vi "Tag_settings_load.vi"(8 "error in (no error)":errorcluster, 10 "PresetName":string, 11 "Gviewer in":refnum<class "Gviewer.lvclass">) -> (0 "error out":errorcluster, 3 "Gviewer out":refnum<class "Gviewer.lvclass">)   [LabVIEW 2020, in "Sgraph_lib_V1.lvlib" / "Gviewer.lvclass"]
doc: "Andre Koelewijn, 5 feb 2021\n\nLoad presets for one of the Viewports"
uses:
  Gviewer.lvclass
  controls/Typedef-PresetFileFormat.ctl
  controls/EditTagOneTag.ctl
  Gviewer.lvclass/Gviewer.ctl
  controls/Typedef_SelProperties.ctl
  controls/Typedef_LineType.ctl
  controls/Typedef_Live.ctl
panel:
  out "value":T1 {"PresetSave"."Presets"."max" format="%#_3p"; "PresetSave"."Presets"."min" format="%#_3p"}
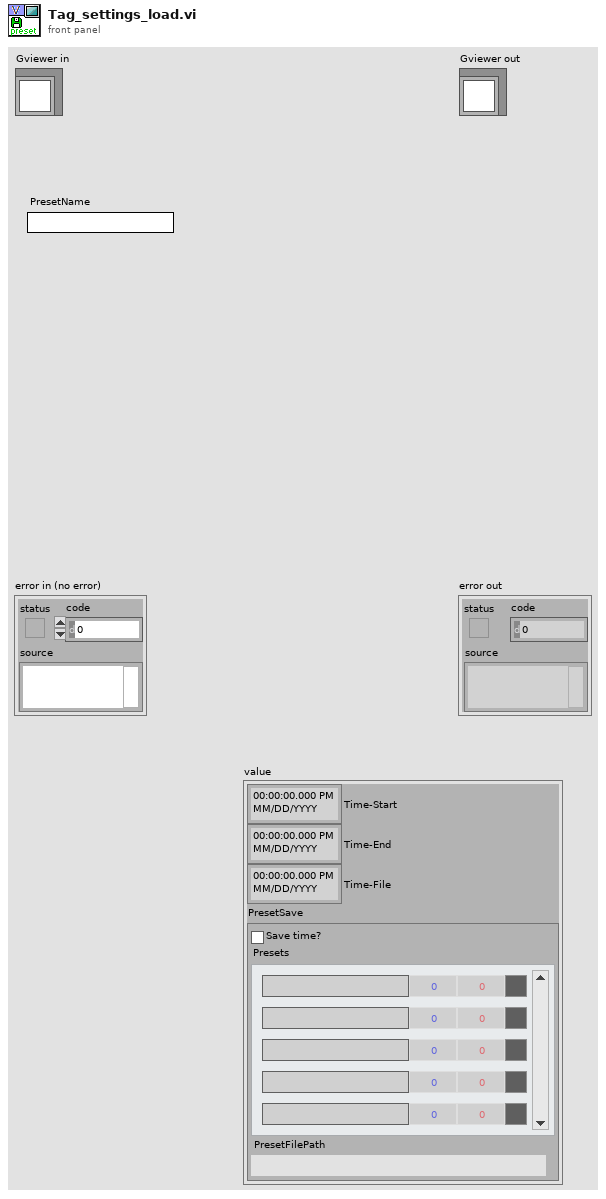
[diagram p1: front panel]
types:
  T1 = typedef "Sgraph_lib_V1.lvlib/Gviewer.lvclass/Typedef-PresetFileFormat.ctl" = cluster{"Time-Start":timestamp, "Time-End":timestamp, "Time-File":timestamp, "PresetSave":cluster{"Save time?":bool, "Presets":T2[], "PresetFilePath":path}}
  T2 = typedef "Sgraph_lib_V1.lvlib/Gviewer.lvclass/EditTagOneTag.ctl" = cluster{"TAG":string, "min":dbl, "max":dbl, "Color":u32}
  T3 = enum16{"big-endian, network order", "native, host order", "little-endian"}
  T4 = typedef "Sgraph_lib_V1.lvlib/Gviewer.lvclass/Typedef_Live.ctl" = enum16{"Live View", "Freeze"}
  T5 = typedef "Sgraph_lib_V1.lvlib/Gviewer.lvclass/Typedef_LineType.ctl" = enum16{"num_bare", "num_MinMax_Area", "num_MinMax_Lines", "num_MinMax_Forfor", "num_Max_Area", "num_Max_Line", "num_Max_Forfor", "num_Min_Area", "num_Min_Line", "num_Min_Fosfor", "Boolean_Line_01", "Boolean_Area_01", "Boolean_Fosfor_01", "Boolean_Line_TF", "Boolean_Area_TF", "Boolean_Fosfor_TF", "Boolean_OnOff_Line", "Boolean_OnOff_Area", "Boolean_OnOff_Fosfor", "Boolean_spare", "StringEvent_Line", "StringEvent_TimeLine"}
  T6 = typedef "Sgraph_lib_V1.lvlib/Gviewer.lvclass/Typedef_SelProperties.ctl" = cluster{"Color":u32, "LineType":T5, "max":dbl, "min":dbl}
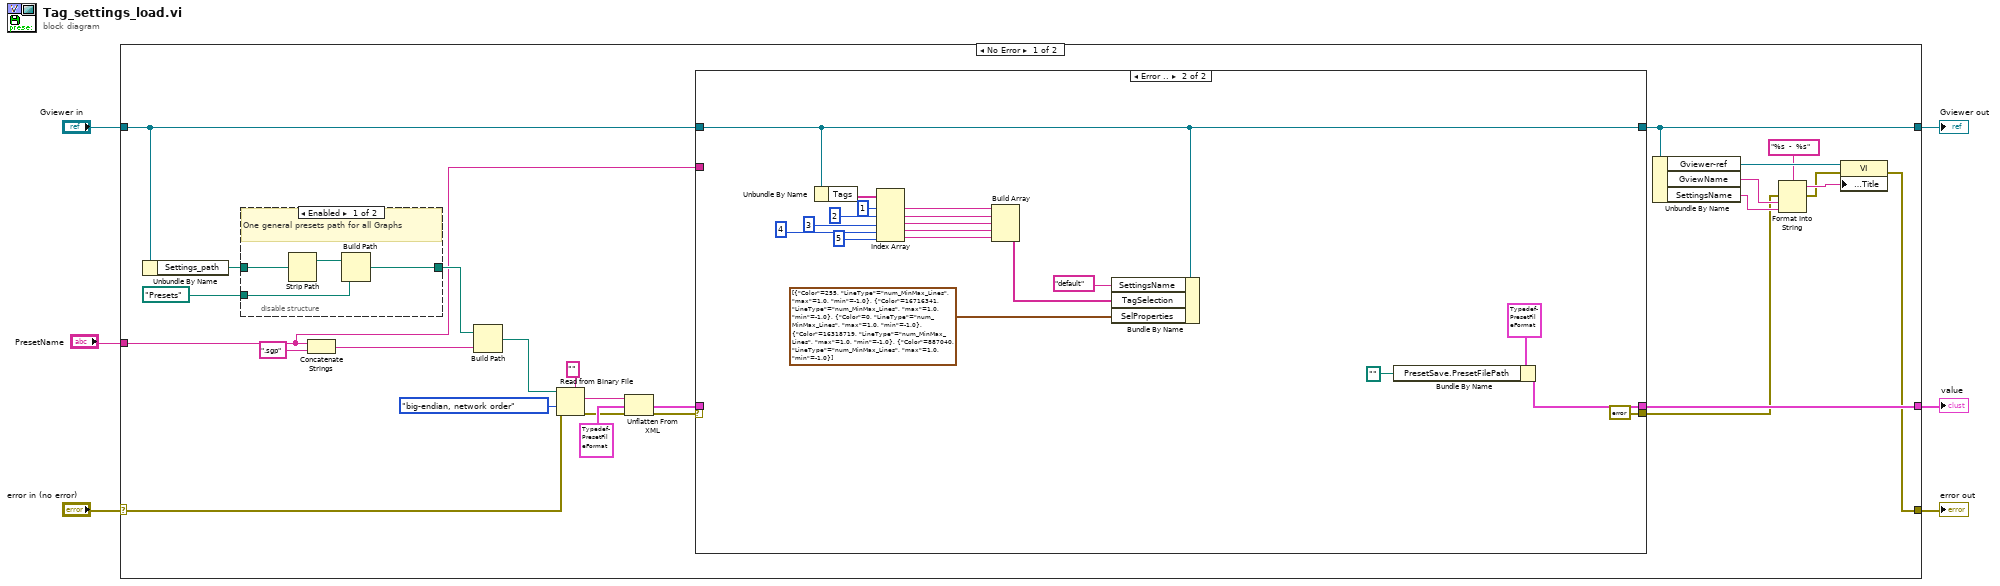
[diagram p0: block diagram]
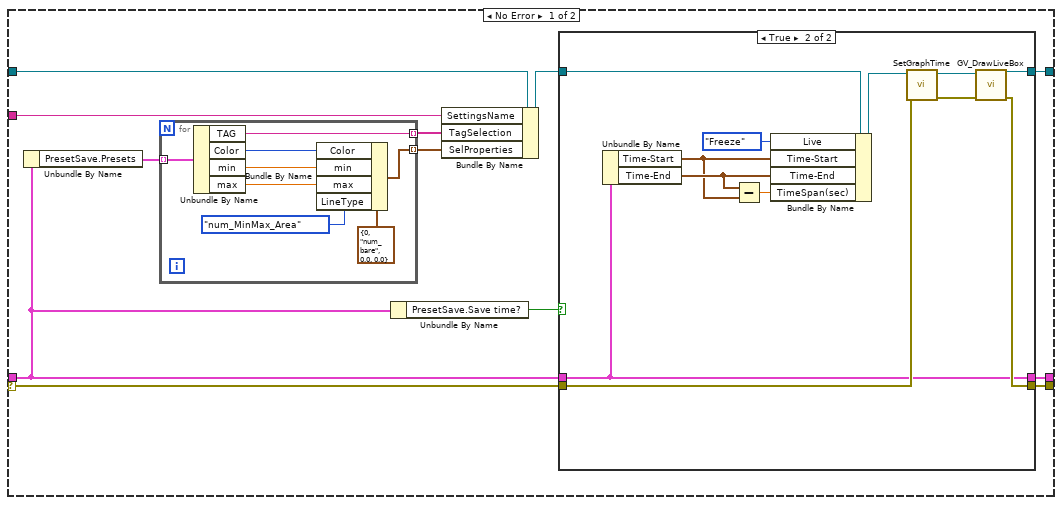
[diagram p2: hidden frame]
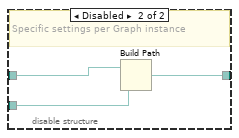
[diagram p4: hidden frame]
diagram:
  n1 = case shown="No Error" "error in (no error)" {
    selector: "error in (no error)" -> [w26 w95]
    tunnel: [w7 w95] -> w5
    tunnel: [w15 w94] -> w3
    tunnel: "Gviewer in" -> [w17 w94]
    tunnel: "PresetName" -> [w16 _]
    tunnel: [w18 _] -> w1
    frame No Error {
      n2 = Unbundle By Name(w17) -> ("Settings_path"=w30:path)
      n3 = disable-structure shown="Enabled" {
        disable-tunnel: w30 -> [w90 w91]
        disable-tunnel: path "Presets" ("name or relative path") -> [w88 w93]
        disable-tunnel: [w87 w92] -> w28
        frame Enabled {
          # "One general presets path for all Graphs"
          n4 = Strip Path(path=w90) -> (stripped path=w89:path)  [unwired: 1 out]
          n5 = Build Path(base path=w89, name or relative path=w88) -> (appended path=w87:path)
        }
        frame Disabled {
          # "Specific settings per Graph instance"
          n6 = Build Path(base path=w91, name or relative path=w93) -> (appended path=w92:path)
        }
      }
      n7 = Concatenate Strings(w16, ".sgp" ("string")) -> (w32:string)
      n8 = Build Path(base path=w28, name or relative path=w32) -> (appended path=w27:path)
      n9 = Read from Binary File(5:"", 8:w26, 9:T3."big-endian, network order" ("byte order (0:big-endian, network order)"), 11:w27) -> (0:w21:errorcluster, 2:w23:string)  [unwired: 2 in, 2 out]
      n10 = Unflatten From XML(xml string=w23, type=T1 {"Time-Start"=timestamp(0 s since 1904-01-01), "Time-End"=timestamp(0 s since 1904-01-01), "Time-File"=timestamp(0 s since 1904-01-01), "PresetSave"={"Save time?"=FALSE, "Presets"=[], "PresetFilePath"=path ""}} ("PresetFileFormat"), error in (no error)=w21) -> (value=w19:T1, error out=w20:errorcluster)
      n11 = case shown="Error .." w20 {
        selector: w20 -> [w34 _]
        tunnel: [w33 errorcluster {"status"=FALSE, "code"=0, "source"=""} ("error out")] -> w8
        tunnel: w19 -> [w36 _]
        tunnel: [w35 w69] -> w18
        tunnel: w17 -> [w44 w68]
        tunnel: [w37 w68] -> w15
        tunnel: w16 -> [w43 _]
        frame No Error {
          n12 = Unbundle By Name(w36) -> ("PresetSave.Presets"=w42:T2[])
          n13 = for {
            tunnel: w42 -> [w67] mode=indexing
            tunnel: [w66] -> w41 mode=indexing
            tunnel: [w60] -> w40 mode=indexing
            n14 = Unbundle By Name(w67) -> ("TAG"=w66:string, "Color"=w64:u32, "min"=w63:dbl, "max"=w62:dbl)
            n15 = Bundle By Name(cluster=T6 {"Color"=0, "LineType"=enum."num_bare", "max"=0.0, "min"=0.0} ("SelProperties"), "Color"=w64, "min"=w63, "max"=w62, "LineType"=Typedef_LineType."num_MinMax_Area") -> (w60:T6)
          }
          n16 = Unbundle By Name(w36) -> ("PresetSave.Save time?"=w39:bool)
          n17 = Bundle By Name(cluster=w44, "SettingsName"=w43, "TagSelection"=w41, "SelProperties"=w40) -> (w38:refnum<class "Gviewer.lvclass">)
          n18 = case shown="True" w39 {
            tunnel: w38 -> [w47 w55]
            tunnel: [w47 w54] -> w37
            tunnel: w36 -> [w46 w51]
            tunnel: [w46 w51] -> w35
            tunnel: w34 -> [w45 w52]
            tunnel: [w45 w53] -> w33
            frame False {
            }
            frame True {
              n19 = Unbundle By Name(w51) -> ("Time-Start"=w49:timestamp, "Time-End"=w50:timestamp)
              n20 = Subtract(x=w50, y=w49) -> (x-y=w48:dbl)
              n21 = Bundle By Name(cluster=w55, "Live"=Typedef_Live."Freeze", "Time-Start"=w49, "Time-End"=w50, "TimeSpan(sec)"=w48) -> (w57:refnum<class "Gviewer.lvclass">)
              n22 = call "SetGraphTime.vi"("error in (no error)"=w52, "Gviewer in"=w57) -> ("error out"=w59:errorcluster, "Gviewer out"=w58:refnum<class "Gviewer.lvclass">)  [unwired: 8 in]
              n23 = call "GV_DrawLiveBox.vi"("error in (no error)"=w59, "Gviewer in"=w58) -> ("error out"=w53:errorcluster, "Gviewer out"=w54:refnum<class "Gviewer.lvclass">)  [unwired: 8 in]
            }
          }
        }
        frame Error {
          n24 = Unbundle By Name(w68) -> ("Tags"=w86:string[])
          n25 = Index Array(array=w86, index #1=1 ("index"), index #2=2 ("index"), index #3=3 ("index"), index #4=4 ("index"), index #5=5 ("index")) -> (element #1=w80:string, element #2=w79:string, element #3=w78:string, element #4=w77:string, element #5=w76:string)
          n26 = Build Array(w80, w79, w78, w77, w76) -> (w74:string[])
          n27 = Bundle By Name(cluster=w68, "SettingsName"="default", "TagSelection"=w74, "SelProperties"=T6[] [{"Color"=255, "LineType"=enum."num_MinMax_Lines", "max"=1.0, "min"=-1.0}, {"Color"=16716341, "LineType"=enum."num_MinMax_Lines", "max"=1.0, "min"=-1.0}, {"Color"=0, "LineType"=enum."num_MinMax_Lines", "max"=1.0, "min"=-1.0}, {"Color"=16318719, "LineType"=enum."num_MinMax_Lines", "max"=1.0, "min"=-1.0}, {"Color"=887040, "LineType"=enum."num_MinMax_Lines", "max"=1.0, "min"=-1.0}]) -> ()  [unwired: 1 out]
          n28 = Bundle By Name(cluster=T1 {"Time-Start"=timestamp(0 s since 1904-01-01), "Time-End"=timestamp(0 s since 1904-01-01), "Time-File"=timestamp(0 s since 1904-01-01), "PresetSave"={"Save time?"=FALSE, "Presets"=[], "PresetFilePath"=path ""}} ("PresetFileFormat"), "PresetSave.PresetFilePath"=path "") -> (w69:T1)
        }
      }
      n29 = Unbundle By Name(w15) -> ("Gviewer-ref"=w14:refnum<vi>, "GviewName"=w12:string, "SettingsName"=w11:string)
      n30 = Format Into String(format string="%s  -  %s", error in=w8, w12, w11) -> (resulting string=w10:string, error out=w9:errorcluster)  [unwired: 1 in]
      n31 = property class="VI"(reference=w14, error in=w9, "Front Panel.Title"=w10) -> (error out=w7:errorcluster)  [unwired: 1 out]
    }
    frame Error {
    }
  }
  "error out" <- w5
  "Gviewer out" <- w3
  "value" <- w1
